vi "Decrement PtByPt.vi"(2 "initialize":bool, 3 "activate":bool, 4 "start":u32) -> (0 "zero crossing":bool, 1 "counter":u32)   [LabVIEW 2020, in "NI_PtbyPt.lvlib"]
doc: "Begins at <B>start</B> and decrements <B>counter</B> by one each time the VI is called when <B>activate</B> is set to TRUE."
uses:
  NI_PtbyPt.lvlib
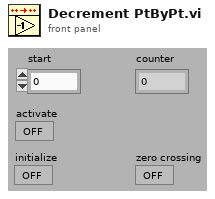
[diagram p1: front panel]
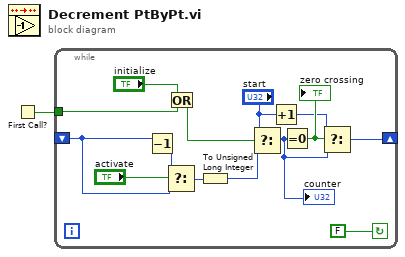
[diagram p0: block diagram]
diagram:
  n1 = First Call?() -> (First Call?: T/F=w1:bool)
  n2 = while {
    tunnel: w1 -> [w3]
    shift-left: _ -> [w12]
    shift-right: [w8] -> _
    stop <- FALSE continue-if-true
    n3 = Decrement(x=w12) -> (x-1=w14:u32)
    n4 = Select(t=w14, s="activate", f=w12) -> (s? t:f=w13:u32)
    n5 = Or(x="initialize", y=w3) -> (x .or. y?=w2:bool)
    n6 = To Unsigned Long Integer(number=w13) -> (unsigned 32bit integer=w11:u32)
    n7 = Select(t="start", s=w2, f=w11) -> (s? t:f=w7:u32)
    "counter" <- w7
    n8 = Increment(x="start") -> (x+1=w6:u32)
    n9 = Equal To 0?(x=w7) -> (x = 0?=w10:bool)
    "zero crossing" <- w10
    n10 = Select(t=w6, s=w10, f=w7) -> (s? t:f=w8:u32)
  }
